vi "DAQParameters.vi"(4 "DAQ Controls":T1={"Minimum Value"=-10.0, "Maximum Value"=10.0, "Physical Channel"="Dev1/ao0", "DAQ Fs (S/s)"=10000.0}, 7 "DAQ Device IN":T2={"DAQ Fs (S/s)"=10000.0, "task"="", "error"={"status"=FALSE, "code"=0, "source"=""}, "Min Value"=-10.0, "Max Value"=10.0}) -> (2 "En Funcionamiento?":bool, 3 "DAQ Device OUT":T2)   [LabVIEW 2010]
uses:
  <vilib>/Utility/error.llb/DialogType.ctl
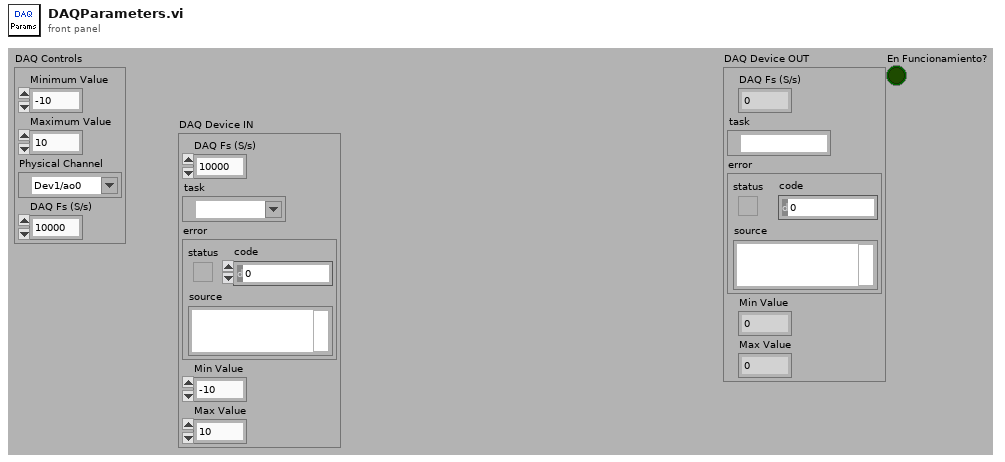
[diagram p1: front panel]
types:
  T1 = cluster{"Minimum Value":dbl, "Maximum Value":dbl, "Physical Channel":tag, "DAQ Fs (S/s)":dbl}
  T2 = cluster{"DAQ Fs (S/s)":dbl, "task":refnum<k21>, "error":errorcluster, "Min Value":dbl, "Max Value":dbl}
  T3 = typedef "DialogType.ctl" = u16
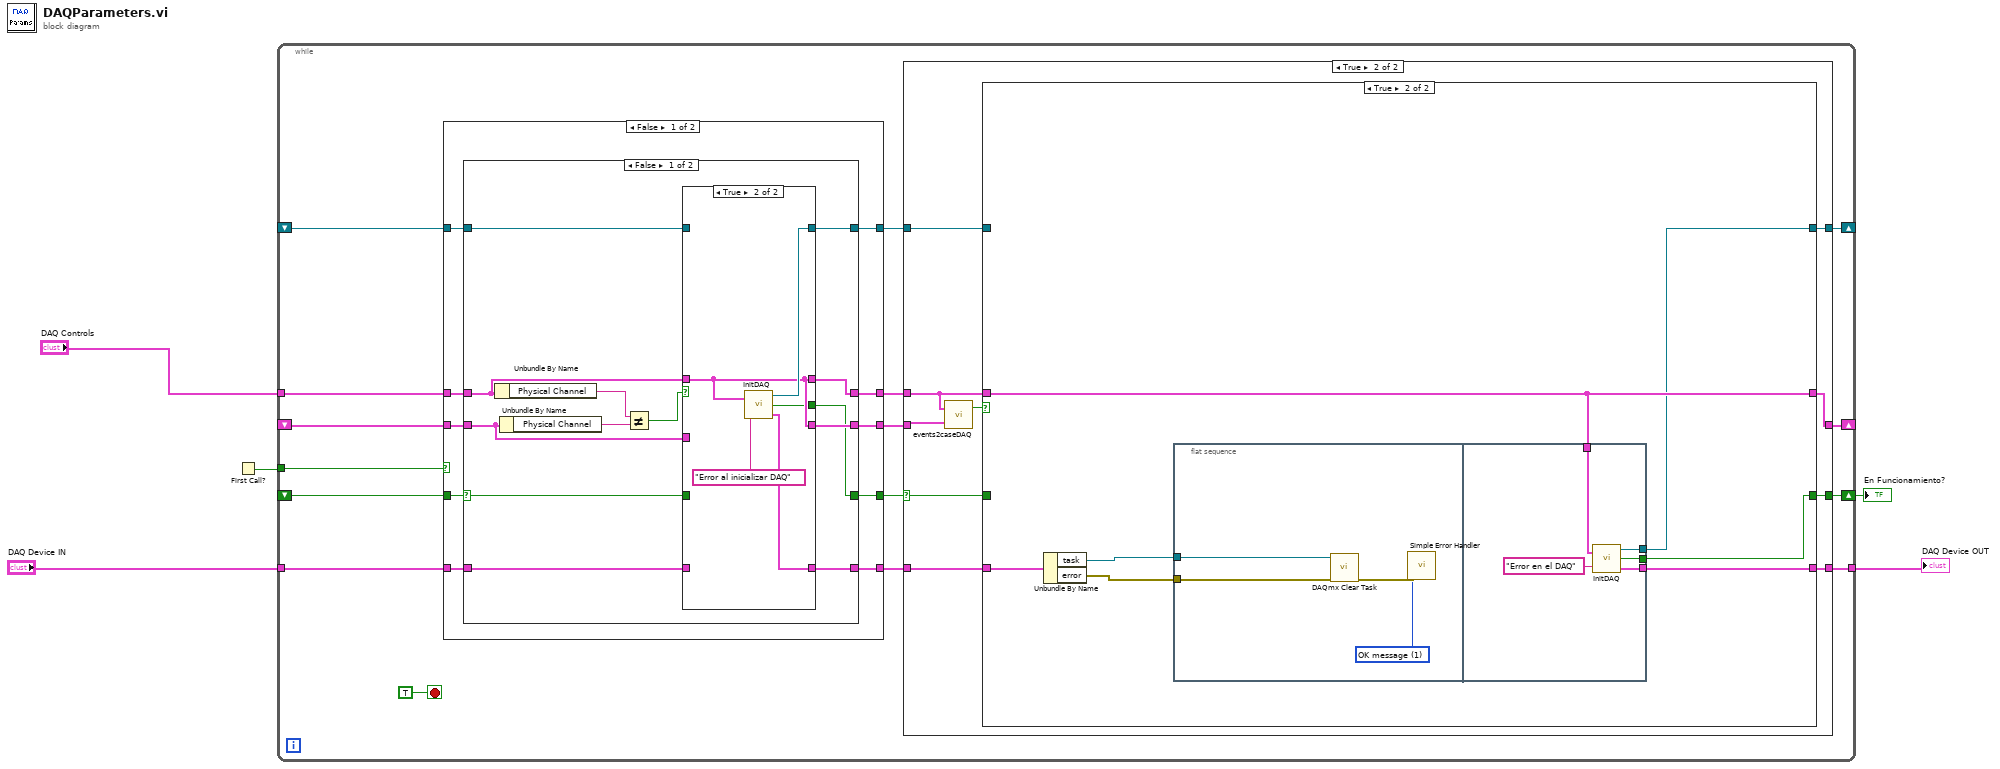
[diagram p0: block diagram]
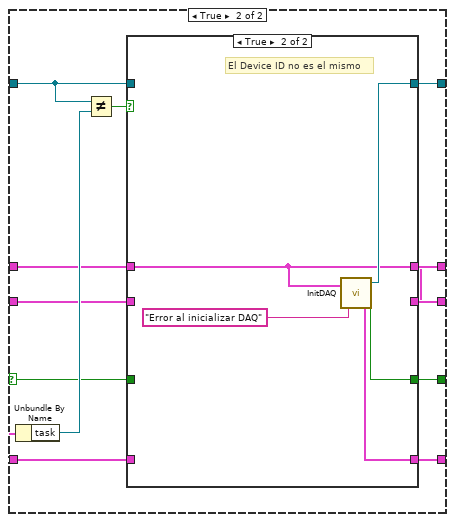
[diagram p3: hidden frame]
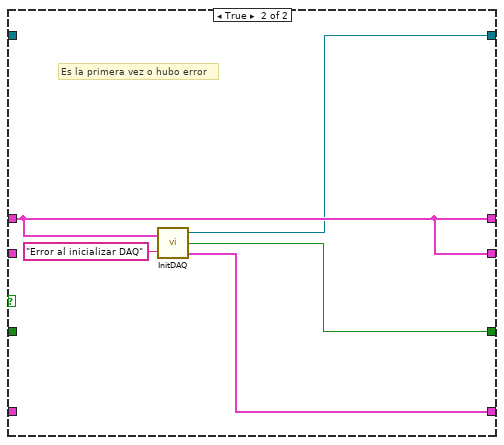
[diagram p5: hidden frame]
diagram:
  n1 = First Call?() -> (First Call?: T/F=w5:bool)
  n2 = while {
    tunnel: "DAQ Controls" -> [w17]
    shift-right: [w20] -> _
    shift-left: _ -> [w16]
    tunnel: "DAQ Device IN" -> [w10]
    tunnel: [w19] -> w3
    tunnel: w5 -> [w6]
    shift-right: [w11] -> _
    shift-left: _ -> [w13]
    shift-right: [w8] -> w2
    shift-left: _ -> [w7]
    stop <- TRUE stop-if-true
    n3 = case shown="False" w6 {
      tunnel: [w26 w78] -> w12
      tunnel: [w28 w80] -> w18
      tunnel: w17 -> [w29 w80]
      tunnel: w16 -> [w24 _]
      tunnel: [w27 w80] -> w15
      tunnel: [w31 w79] -> w14
      tunnel: w10 -> [w30 _]
      tunnel: w13 -> [w23 _]
      tunnel: [w25 w81] -> w9
      tunnel: w7 -> [w22 _]
      frame False {
        n4 = case shown="False" w22 {
          selector: w22 -> [w35 w55]
          tunnel: [w40 w66] -> w31
          tunnel: w30 -> [w33 w65]
          tunnel: w29 -> [w42 w62]
          tunnel: [w39 w61] -> w28
          tunnel: [w38 w60] -> w27
          tunnel: [w41 w59] -> w26
          tunnel: [w37 w58] -> w25
          tunnel: w24 -> [w34 w57]
          tunnel: w23 -> [w32 w56]
          frame False {
            n5 = Unbundle By Name(w42) -> ("Physical Channel"=w44:tag)
            n6 = Unbundle By Name(w34) -> ("Physical Channel"=w43:tag)
            n7 = Not Equal?(x=w44, y=w43) -> (x != y?=w36:bool)
            n8 = case shown="True" w36 {
              tunnel: w42 -> [w49 w52]
              tunnel: [w45 w54] -> w41
              tunnel: [w46 w53] -> w40
              tunnel: [w49 w52] -> w39
              tunnel: [w47 w52] -> w38
              tunnel: [w48 w51] -> w37
              tunnel: w35 -> [w48 _]
              tunnel: w34 -> [w47 _]
              tunnel: w33 -> [w46 _]
              tunnel: w32 -> [w45 _]
              frame False {
              }
              frame True {
                n9 = call "InitDAQ.vi"("message"="Error al inicializar DAQ", "DAQ Parameters"=w52) -> ("DAQ Device OUT"=w53:T2, "Inicializo DAQ?"=w51:bool, "task OUT"=w54:refnum<k21>)
              }
            }
          }
          frame True {
            n10 = Unbundle By Name(w65) -> ("task"=w64:refnum<k21>)
            n11 = Not Equal?(x=w56, y=w64) -> (x != y?=w63:bool)
            n12 = case shown="True" w63 {
              tunnel: [w71 w74] -> w66
              tunnel: w65 -> [w71 _]
              tunnel: w62 -> [w70 w73]
              tunnel: [w70 w73] -> w61
              tunnel: [w69 w73] -> w60
              tunnel: [w67 w76] -> w59
              tunnel: [w68 w75] -> w58
              tunnel: w57 -> [w69 _]
              tunnel: w55 -> [w68 _]
              tunnel: w56 -> [w67 _]
              frame False {
                # "Sigue siendo todo igual"
              }
              frame True {
                # "El Device ID no es el mismo"
                n13 = call "InitDAQ.vi"("message"="Error al inicializar DAQ", "DAQ Parameters"=w73) -> ("DAQ Device OUT"=w74:T2, "Inicializo DAQ?"=w75:bool, "task OUT"=w76:refnum<k21>)
              }
            }
          }
        }
      }
      frame True {
        # "Es la primera vez o hubo error"
        n14 = call "InitDAQ.vi"("message"="Error al inicializar DAQ", "DAQ Parameters"=w80) -> ("DAQ Device OUT"=w79:T2, "Inicializo DAQ?"=w81:bool, "task OUT"=w78:refnum<k21>)
      }
    }
    n15 = case shown="True" w9 {
      selector: w9 -> [w82 w87]
      tunnel: [w85 w94] -> w20
      tunnel: [w84 w93] -> w19
      tunnel: w12 -> [w83 w92]
      tunnel: w18 -> [w85 w86]
      tunnel: w15 -> [_ w89]
      tunnel: w14 -> [w84 w91]
      tunnel: [w83 w90] -> w11
      tunnel: [w82 w88] -> w8
      frame False {
      }
      frame True {
        n16 = call "events2caseDAQ.vi"("DAQ Controls Old"=w89, "DAQ Controls New"=w86) -> ("DAQ Cambio?"=w95:bool)  [unwired: 1 out]
        n17 = case shown="True" w95 {
          tunnel: [w99 w103] -> w94
          tunnel: w86 -> [w99 w103]
          tunnel: w91 -> [w98 w106]
          tunnel: [w98 w100] -> w93
          tunnel: w92 -> [w97 _]
          tunnel: [w97 w102] -> w90
          tunnel: [w96 w101] -> w88
          tunnel: w87 -> [w96 _]
          frame False {
          }
          frame True {
            n18 = Unbundle By Name(w106) -> ("task"=w104:refnum<k21>, "error"=w105:errorcluster)
            n19 = flat-sequence {
              tunnel: w104 -> [w108]
              tunnel: w105 -> [w107]
              tunnel: w103 -> [w114]
              tunnel: [w113] -> w102
              tunnel: [w112] -> w101
              tunnel: [w111] -> w100
              frame #0 {
                w109 = T3 1 items=["no dialog", "OK message", "continue or stop message", "OK message + warnings", "continue/stop + warnings"] ("type of dialog (OK msg:1)")
                n20 = call <vilib>:"DAQmx Clear Task.vi"("task in"=w108, "error in"=w107) -> ("error out"=w110:errorcluster)  [unwired: 13 in]
                n21 = call <vilib>:"Simple Error Handler.vi"("type of dialog (OK msg:1)"=w109, "error in (no error)"=w110) -> ()  [unwired: 3 in, 5 out]
              }
              frame #1 {
                n22 = call "InitDAQ.vi"("message"="Error en el DAQ", "DAQ Parameters"=w114) -> ("DAQ Device OUT"=w111:T2, "Inicializo DAQ?"=w112:bool, "task OUT"=w113:refnum<k21>)
              }
            }
          }
        }
      }
    }
  }
  "DAQ Device OUT" <- w3
  "En Funcionamiento?" <- w2
